vi "Replase ALR_checks.vi"(9 "ALR_CHK":bool[](array[boolean]), 10 "N_start (0)":i32, 11 "ALR_ON_OFF in":T1) -> (3 "ALR_ON_OFF out":T1)   [LabVIEW 2019]
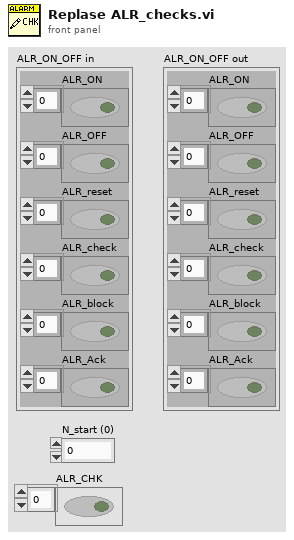
[diagram p1: front panel]
types:
  T1 = cluster{"ALR_ON":bool[], "ALR_OFF":bool[], "ALR_reset":bool[], "ALR_check":bool[], "ALR_block":bool[], "ALR_Ack":bool[]}
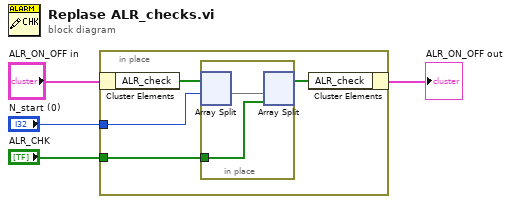
[diagram p0: block diagram]
diagram:
  n1 = in-place {
    in-place-border: "ALR_CHK" -> [w6]
    in-place-border: "N_start (0)" -> [w5]
    n2 = in-place-cluster #1("ALR_ON_OFF in") -> ("ALR_check"=w8:bool[])
    n3 = in-place {
      in-place-border: w6 -> [w9]
      n4 = in-place-split #2(w8, w5) -> (w10:bool[])  [unwired: 1 out]
      n5 = in-place-split #2(w10, w9) -> (w7:bool[])  [unwired: 1 out]
    }
    n6 = in-place-cluster #1("ALR_check"=w7) -> (→"ALR_ON_OFF out":T1)
  }
